vi "To Pretty String (Numeric).vi"(0 "Variant in":variant, 5 "indent":i32, 7 "enable LabVIEW extensions? (T)":bool=TRUE, 11 "error in (no error)":errorcluster) -> (4 "String":string, 15 "error out":errorcluster)   [LabVIEW 2020, in "Variant JSON API.lvlib"]
doc: "Flattens the given JSON data to a string."
uses:
  Variant JSON API.lvlib
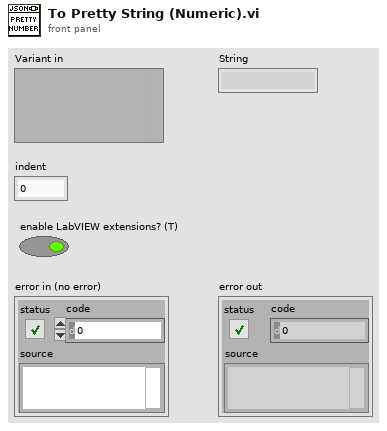
[diagram p1: front panel]
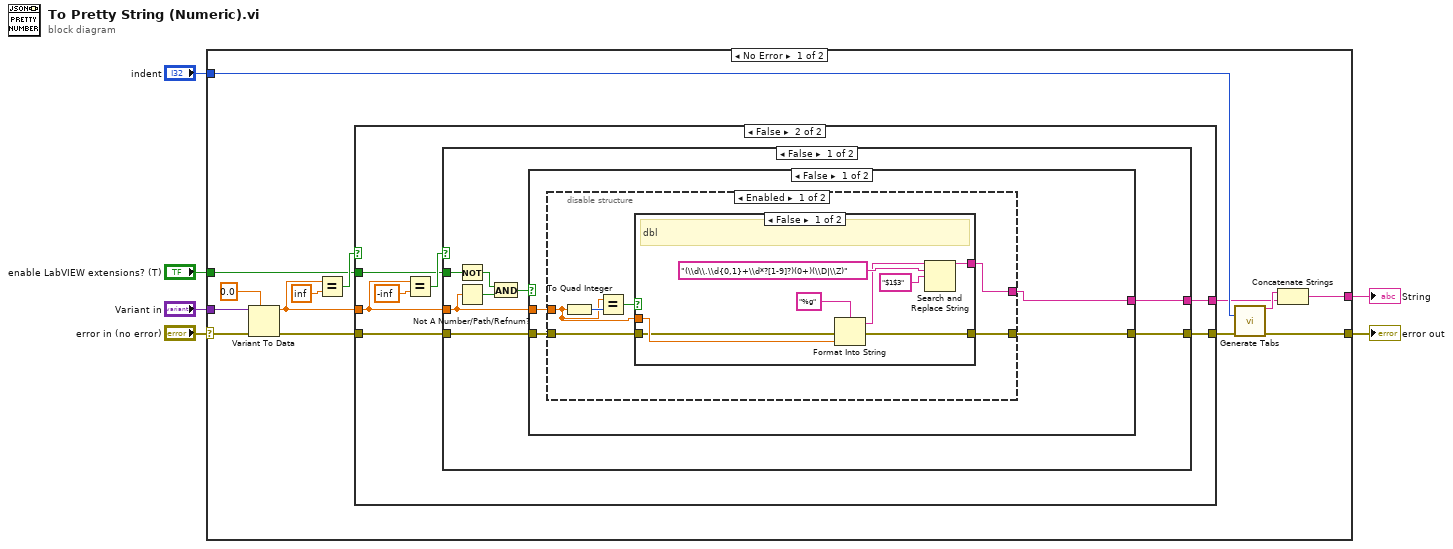
[diagram p0: block diagram]
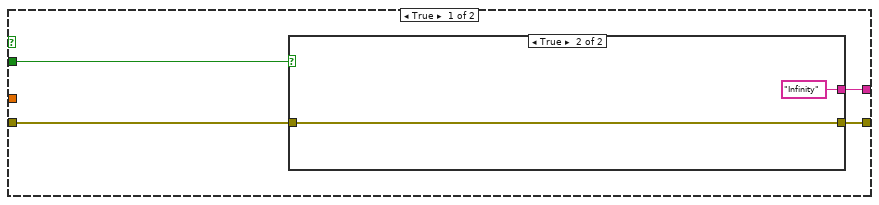
[diagram p2: hidden frame]
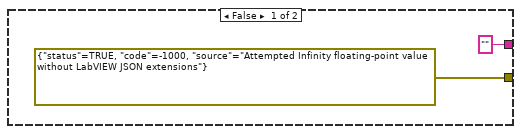
[diagram p3: hidden frame]
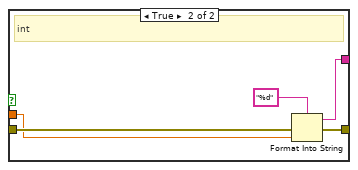
[diagram p4: hidden frame]
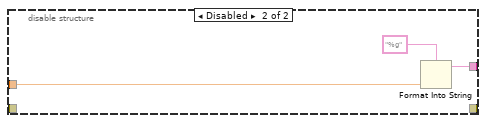
[diagram p5: hidden frame]
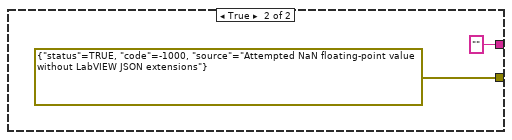
[diagram p6: hidden frame]
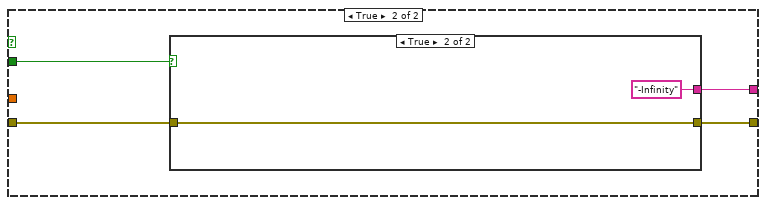
[diagram p7: hidden frame]
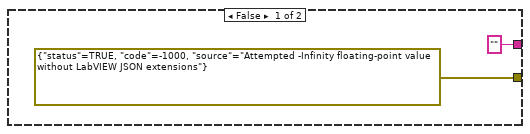
[diagram p8: hidden frame]
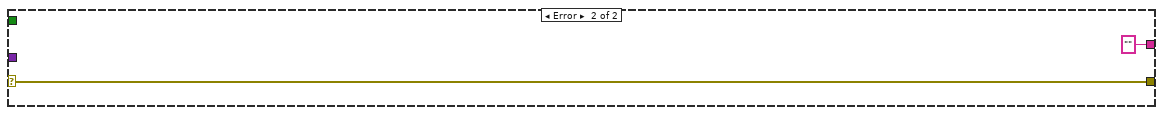
[diagram p9: hidden frame]
diagram:
  n1 = case shown="No Error" "error in (no error)" {
    selector: "error in (no error)" -> [w20 w81]
    tunnel: "Variant in" -> [w7 _]
    tunnel: [w9 ""] -> w4
    tunnel: [w8 w81] -> w3
    tunnel: "enable LabVIEW extensions? (T)" -> [w17 _]
    tunnel: "indent" -> [w13 _]
    frame No Error {
      n2 = Variant To Data(error in=w20, type=0.0 ("y"), Variant=w7) -> (data=w15:dbl, error out=w16:errorcluster)
      n3 = Equal?(x=w15, y=inf) -> (x = y?=w18:bool)
      n4 = case shown="False" w18 {
        tunnel: w16 -> [w22 w35]
        tunnel: [w24 w34] -> w10
        tunnel: [w21 w33] -> w12
        tunnel: w15 -> [_ w31]
        tunnel: w17 -> [w23 w29]
        frame True {
          n5 = case shown="True" w23 {
            tunnel: ["" "Infinity"] -> w24
            tunnel: w22 -> [_ w27]
            tunnel: [errorcluster {"status"=TRUE, "code"=-1000, "source"="Attempted Infinity floating-point value without LabVIEW JSON extensions"} ("error IO") w27] -> w21
            frame False {
            }
            frame True {
            }
          }
        }
        frame False {
          n6 = Equal?(x=w31, y=-inf) -> (x = y?=w30:bool)
          n7 = case shown="False" w30 {
            tunnel: w35 -> [w43 w73]
            tunnel: [w42 w74] -> w34
            tunnel: [w41 w75] -> w33
            tunnel: w31 -> [w37 _]
            tunnel: w29 -> [w39 w72]
            frame False {
              n8 = Not(x=w39) -> (.not. x?=w38:bool)
              n9 = Not A Number/Path/Refnum?(number/path/refnum=w37) -> (NaN/Path/Refnum?=w36:bool)
              n10 = And(x=w38, y=w36) -> (x .and. y?=w40:bool)
              n11 = case shown="False" w40 {
                tunnel: w43 -> [w47 _]
                tunnel: [w46 ""] -> w42
                tunnel: [w45 errorcluster {"status"=TRUE, "code"=-1000, "source"="Attempted NaN floating-point value without LabVIEW JSON extensions"} ("error IO")] -> w41
                tunnel: w37 -> [w44 _]
                frame False {
                  n12 = disable-structure shown="Enabled" {
                    disable-tunnel: w47 -> [w52 _]
                    disable-tunnel: [w51 w68] -> w46
                    disable-tunnel: [w50 _] -> w45
                    disable-tunnel: w44 -> [w48 w69]
                    frame Enabled {
                      n13 = To Quad Integer(1:w48) -> (0:w49:i64)
                      n14 = Equal?(x=w48, y=w49) -> (x = y?=w53:bool)
                      n15 = case shown="False" w53 {
                        tunnel: w52 -> [w59 w64]
                        tunnel: w48 -> [w61 w62]
                        tunnel: [w54 w65] -> w51
                        tunnel: [w58 w63] -> w50
                        frame False {
                          # "dbl"
                          n16 = Format Into String(format string="%g", error in=w59, w61) -> (resulting string=w55:string, error out=w58:errorcluster)  [unwired: 1 in]
                          n17 = Search and Replace String(input string=w55, search string="(\\d\\.\\d{0,1}+\\d*?[1-9]?)(0+)(\\D|\\Z)", replace string="$1$3" ("replace string (\"\")")) -> (result string=w54:string)  [unwired: 5 in, 3 out]
                        }
                        frame True {
                          # "int"
                          n18 = Format Into String(format string="%d", error in=w64, w62) -> (resulting string=w65:string, error out=w63:errorcluster)  [unwired: 1 in]
                        }
                      }
                    }
                    frame Disabled {
                      n19 = Format Into String(format string="%g", w69) -> (resulting string=w68:string)  [unwired: 2 in, 1 out]
                    }
                  }
                }
                frame True {
                }
              }
            }
            frame True {
              n20 = case shown="True" w72 {
                tunnel: ["" "-Infinity"] -> w74
                tunnel: w73 -> [_ w78]
                tunnel: [errorcluster {"status"=TRUE, "code"=-1000, "source"="Attempted -Infinity floating-point value without LabVIEW JSON extensions"} ("error IO") w78] -> w75
                frame False {
                }
                frame True {
                }
              }
            }
          }
        }
      }
      n21 = call "Generate Tabs.vi"("indent"=w13, "error in (no error)"=w12) -> ("Tabs"=w11:string, "error out"=w8:errorcluster)  [unwired: 12 in]
      n22 = Concatenate Strings(w11, w10) -> (w9:string)
    }
    frame Error {
    }
  }
  "String" <- w4
  "error out" <- w3
